vi "ParseArguments.vi"(8 "error in (no error)":errorcluster, 9 "Inputs":string[](array[string]), 11 "SetConditionalSymbol in":refnum<class "SetConditionalSymbol.lvclass">) -> (0 "error out":errorcluster, 3 "SetConditionalSymbol out":refnum<class "SetConditionalSymbol.lvclass">)   [LabVIEW 2014, in "SetConditionalSymbol.lvclass"]
uses:
  SetConditionalSymbol.lvclass
  <nishared>/LabVIEW CLI/Operations/Utilities/OperationErrorType.ctl
  SetConditionalSymbol.lvclass/SetConditionalSymbol.ctl
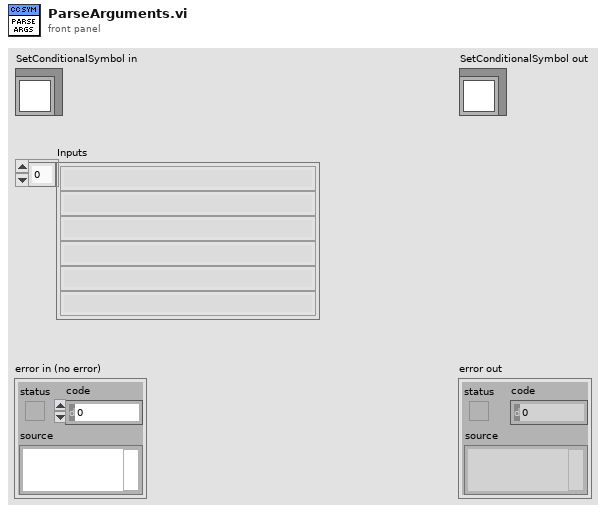
[diagram p1: front panel]
types:
  T1 = typedef "OperationErrorType.ctl" = enum16{"RequiredArgumentMissing", "UnknownArguments", "LoggerSetMultipleTimes", "OperationBrokenError"}
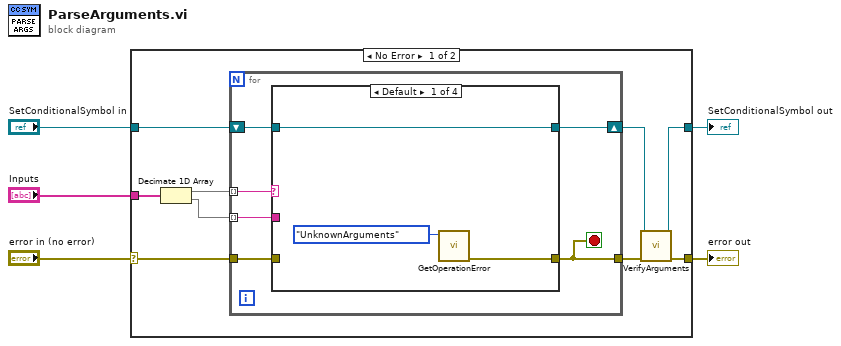
[diagram p0: block diagram]
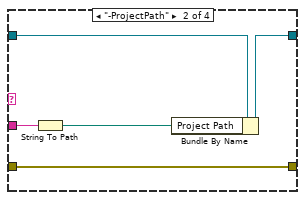
[diagram p2: hidden frame]
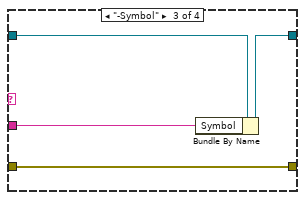
[diagram p3: hidden frame]
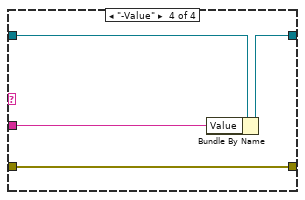
[diagram p4: hidden frame]
diagram:
  n1 = case shown="No Error" "error in (no error)" {
    selector: "error in (no error)" -> [w10 w38]
    tunnel: [w8 w38] -> w4
    tunnel: [w6 w37] -> w2
    tunnel: "SetConditionalSymbol in" -> [w13 w37]
    tunnel: "Inputs" -> [w14 _]
    frame No Error {
      n2 = Decimate 1D Array(w14) -> (w12:string[], w11:string[])
      n3 = for {
        shift-right: [w19] -> w7
        shift-left: w13 -> [w20]
        tunnel: w12 -> [w18] mode=indexing
        tunnel: w11 -> [w17] mode=indexing
        tunnel: w10 -> [w16]
        tunnel: [w15] -> w9
        stop <- w15 stop-if-true
        n4 = case shown="Default" w18 {
          tunnel: w20 -> [w22 w28 w32 w36]
          tunnel: [w22 w26 w30 w34] -> w19
          tunnel: w17 -> [_ w24 w31 w35]
          tunnel: w16 -> [_ w25 w29 w33]
          tunnel: [w21 w25 w29 w33] -> w15
          frame Default {
            n5 = call <nishared>:"GetOperationError.vi"("Operation Error Type"=OperationErrorType."UnknownArguments") -> ("error out"=w21:errorcluster)  [unwired: 10 in]
          }
          frame "-ProjectPath" {
            n6 = String To Path(string=w24) -> (path=w27:path)
            n7 = Bundle By Name(cluster=w28, "Project Path"=w27) -> (w26:refnum<class "SetConditionalSymbol.lvclass">)
          }
          frame "-Symbol" {
            n8 = Bundle By Name(cluster=w32, "Symbol"=w31) -> (w30:refnum<class "SetConditionalSymbol.lvclass">)
          }
          frame "-Value" {
            n9 = Bundle By Name(cluster=w36, "Value"=w35) -> (w34:refnum<class "SetConditionalSymbol.lvclass">)
          }
        }
      }
      n10 = call "VerifyArguments.vi"("error in (no error)"=w9, "SetConditionalSymbol in"=w7) -> ("error out"=w8:errorcluster, "SetConditionalSymbol out"=w6:refnum<class "SetConditionalSymbol.lvclass">)  [unwired: 8 in]
    }
    frame Error {
    }
  }
  "error out" <- w4
  "SetConditionalSymbol out" <- w2
